vi "Counter Example.vi"() -> ()   [LabVIEW 2015]
uses:
  <vilib>/Erdos Miller/LV-VI/Check Out Ref.vi
  <vilib>/Erdos Miller/LV-VI/Check In Ref.vi
  <vilib>/Erdos Miller/LV-Async/async-xnode/LV-Async.xnode
  <vilib>/Erdos Miller/LV-Async/await-xnode/LV-Await.xnode
  <vilib>/Erdos Miller/LV-VI/LV-VI.lvlib
panel:
  in  "Stop":bool
  out "Counter 2":dbl
  out "Counter":dbl
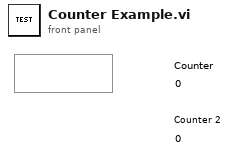
[diagram p1: front panel]
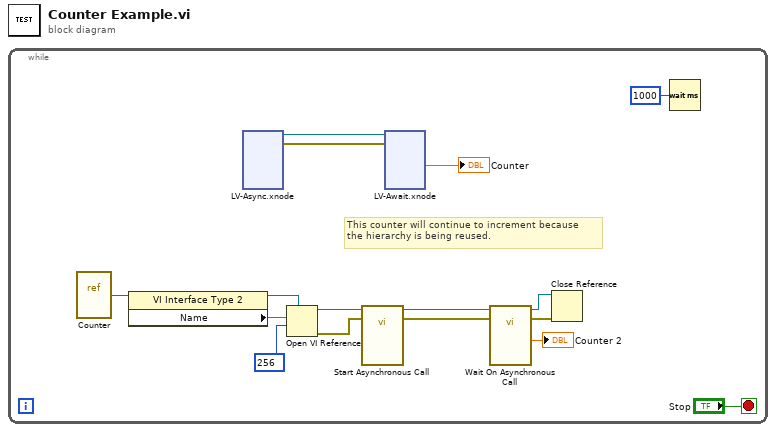
[diagram p0: block diagram]
diagram:
  n1 = while {
    stop <- "Stop" stop-if-true
    # "This counter will continue to increment because\nthe hierarchy is being reused."
    n2 = vi-ref "Counter.vi"() -> (w7:refnum<vi>)
    n3 = property class="VI Interface Type 2"(reference=w7) -> (reference out=w9:refnum<vi>, "Name"=w8:string)  [unwired: 1 in, 1 out]
    n4 = xnode "LV-Async.xnode"() -> ("Error Out"=w3:errorcluster, "VI Ref"=w2:refnum<vi>)  [unwired: 1 in]
    n5 = Open VI Reference(type specifier VI Refnum (for type only)=w9, vi path=w8, options=256) -> (vi reference=w11:refnum<vi>, error out=w12:errorcluster)  [unwired: 3 in]
    n6 = call-by-ref "Start Asynchronous Call"(reference=w11, error in=w12) -> (reference out=w13:refnum<vi>, error out=w14:errorcluster)  [unwired: 11 in, 1 out]
    n7 = xnode "LV-Await.xnode"("Error In"=w3, "VI Ref"=w2) -> ("Counter"=→"Counter":dbl)  [unwired: 1 out]
    n8 = call-by-ref "Wait On Asynchronous Call"(reference=w13, error in=w14) -> (reference out=w16:refnum<vi>, error out=w15:errorcluster, "Counter"=→"Counter 2":dbl)  [unwired: 11 in]
    n9 = Close Reference(reference=w16, error in (no error)=w15) -> ()  [unwired: 1 out]
    n10 = Wait (ms)(milliseconds to wait=u32 1000) -> ()  [unwired: 1 out]
  }
